vi "WPI_CameraGet Image Compression.vi"(8 "error in (no error)":errorcluster, 11 "CameraDevRef":T1={"Camera Address"="192.168.0.90", "CameraStatus"={"status"=FALSE, "code"=0, "source"=""}}) -> (0 "error out":errorcluster, 2 "Compression":i32, 3 "CameraDevRef Out":T1)   [LabVIEW 2017]
doc: "Returns the level of compression of the image from the camera. The higher the level of image compression, the smaller the file size but the lower the image quality.\n\nThis software is licensed. Open the labview\\readme\\WPI Robotics Library Open Source License.txt file for more information."
uses:
  <vilib>/Rock Robotics/WPI/Camera/WPI_CameraDevRef.ctl
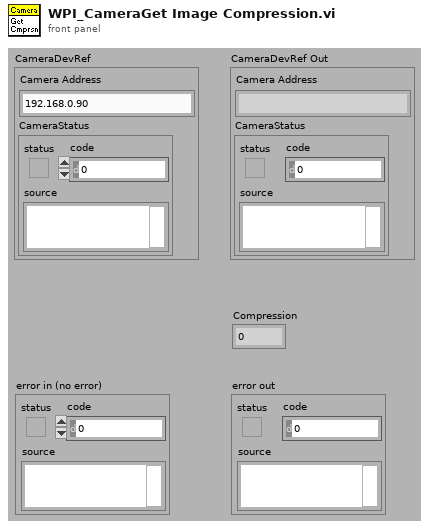
[diagram p1: front panel]
types:
  T1 = typedef "WPI_CameraDevRef.ctl" = cluster{"Camera Address":string, "CameraStatus":errorcluster}
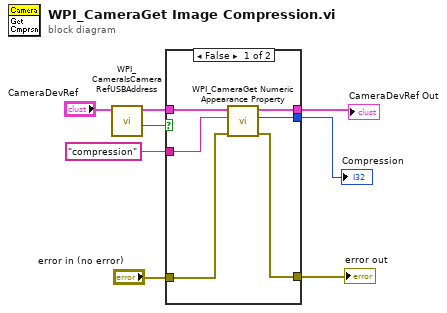
[diagram p0: block diagram]
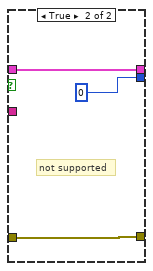
[diagram p2: hidden frame]
diagram:
  n1 = call <vilib>:"WPI_CameraIsCameraRefUSBAddress.vi"("CameraDevRef"="CameraDevRef") -> ("USB?"=w3:bool, "CameraDevRef out"=w2:T1)  [unwired: 7 in, 2 out]
  n2 = case shown="False" w3 {
    tunnel: w2 -> [w14 w17]
    tunnel: [w13 w17] -> w8
    tunnel: "compression" ("Property Name") -> [w12 _]
    tunnel: [w11 0 ("Compression")] -> w6
    tunnel: "error in (no error)" -> [w10 w15]
    tunnel: [w9 w15] -> w4
    frame False {
      n3 = call <vilib>:"WPI_CameraGet Numeric Appearance Property.vi"("error in (no error)"=w10, "Property Name"=w12, "CameraDevRef"=w14) -> ("error out"=w9:errorcluster, "Value"=w11:i32, "CameraDevRef dup"=w13:T1)  [unwired: 6 out]
    }
    frame True {
      # "not supported"
    }
  }
  "CameraDevRef Out" <- w8
  "Compression" <- w6
  "error out" <- w4
